vi "Amplitude Spectrum (sim).vi"() -> ()   [LabVIEW 2020]
doc: "Uses the FFT Spectrum (Mag-Phase) VI to window the signal and display the Amplitude and Phase spectrum. The example also uses the different averaging modes. A subVI simulates a sampled signal."
uses:
  <vilib>/measure/maspectr.llb/FFT Spectrum (Mag-Phase).vi
  <vilib>/measure/NI_MAPro.lvlib
panel:
  in  "sampling info":cluster{"Fs":dbl, "#s":dbl}={"Fs"=51200.0, "#s"=1024.0} {"#s" format="%#.6g"; "Fs" format="%#.6g"}
  in  "signal generator":T1={"type"=enum."Sine Wave", "frequency"=1000.0, "amplitude"=1.0}
  out "averages completed":dbl
  out "Linear averaging done":bool
  in  "Restart averaging":bool
  out "Phase spectrum":cluster{"f0":dbl, "df":dbl, "phase":dbl[]}(graph)
  in  "averaging parameters":T2={"averaging mode"=enum."RMS averaging", "weighting mode"=enum."Exponential", "number of averages"=10} {"number of averages" min=1}
  in  "window":T3(ring)=enum."Hanning"
  out "Amplitude spectrum":cluster{"f0":dbl, "df":dbl, "magnitude":dbl[]}(graph)
  in  "Stop":bool
  # "Overview: Demonstrates using the FFT Spectrum (Mag-Phase) VI to window the signal and display the Amplitude and Phase spectrum.\nRequirements: LabVIEW Full Development System\nInstructions: \n1. Run the VI.\n2. Change the signal generator type, frequency, and amplitude.\n3. Change the averaging parameters to explore various FFT averaging and weighting modes.\n4. Click Stop to stop the VI."
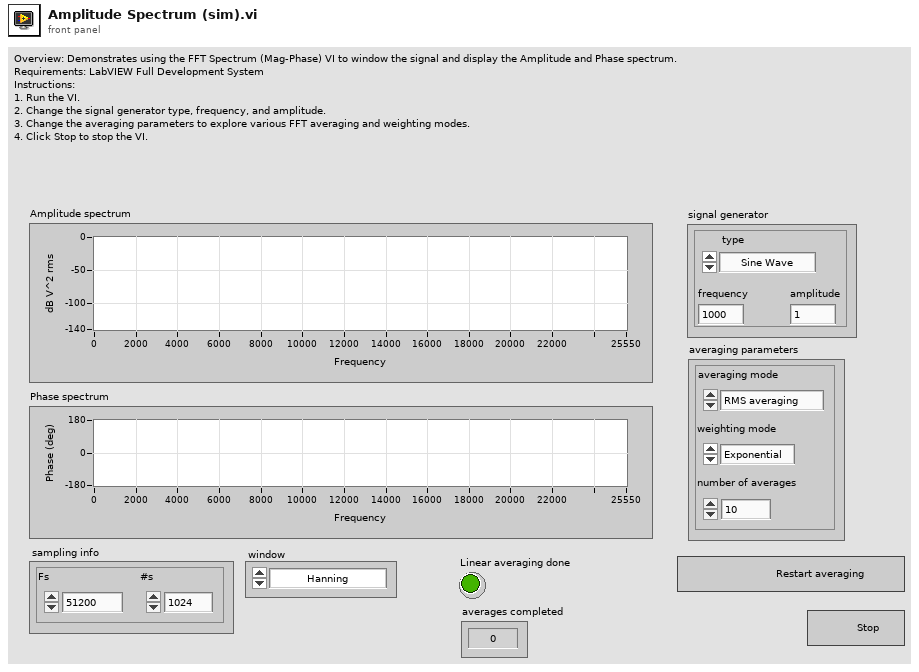
[diagram p1: front panel]
types:
  T1 = cluster{"type":enum16{"Sine Wave", "Triangle Wave", "Square Wave", "Sawtooth Wave"}, "frequency":dbl, "amplitude":dbl}
  T2 = cluster{"averaging mode":enum16{"No averaging", "Vector averaging", "RMS averaging", "Peak hold"}, "weighting mode":enum16{"Linear", "Exponential"}, "number of averages":u32}
  T3 = enum16{"None ", "Hanning", "Hamming", "Blackman-Harris", "Exact Blackman", "Blackman", "Flat Top", "4 Term B-Harris ", "7 Term B-Harris", "Low Sidelobe"}
  T4 = cluster{"dB On (F)":bool, "unwrap phase (F)":bool, "convert to degree (F)":bool}
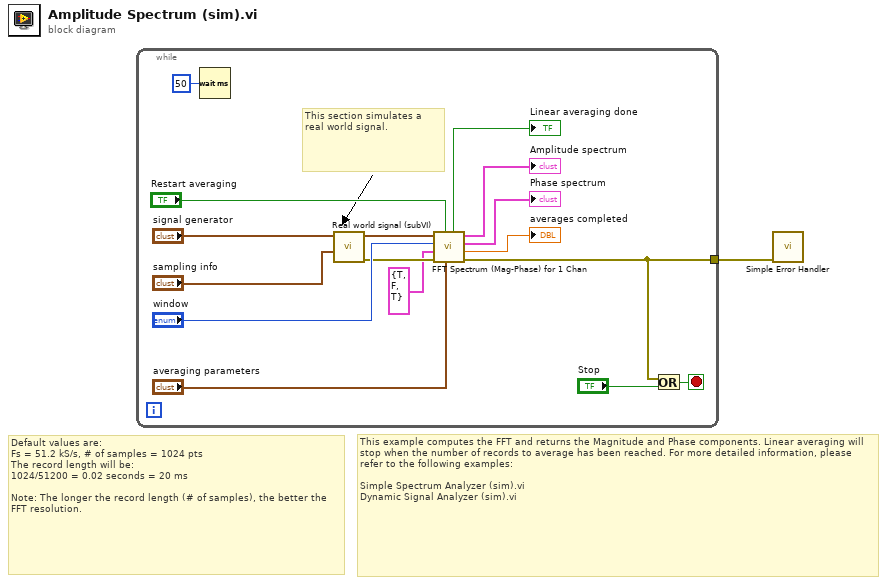
[diagram p0: block diagram]
diagram:
  # "This example computes the FFT and returns the Magnitude and Phase components. Linear averaging will stop when the number of records to average has been reached. For more detailed information, please refer to the following examples:\n\nSimple Spectrum Analyzer (sim).vi\nDynamic Signal Analyzer (sim).vi"
  # "Default values are:\nFs = 51.2 kS/s, # of samples = 1024 pts\nThe record length will be:\n1024/51200 = 0.02 seconds = 20 ms\n\nNote: The longer the record length (# of samples), the better the FFT resolution."
  n1 = while {
    tunnel: [w6] -> w1
    stop <- w7 stop-if-true
    # "This section simulates a real world signal."
    n2 = Wait (ms)(milliseconds to wait=u32 50 ("millisecond multiple")) -> ()  [unwired: 1 out]
    n3 = call "Real world signal (subVI).vi"("sampling info"="sampling info", "signal generator"="signal generator") -> ("error out"=w10:errorcluster, "time signal"=w5:waveform(dbl))  [unwired: 8 in]
    n4 = call-poly <vilib>:"FFT Spectrum (Mag-Phase) for 1 Chan.vi"("averaging parameters"="averaging parameters", "restart averaging (F)"="Restart averaging", "error in (no error)"=w10, "view"=T4 {"dB On (F)"=TRUE, "unwrap phase (F)"=FALSE, "convert to degree (F)"=TRUE}, "window"="window", "time signal"=w5) -> ("error out"=w6:errorcluster, "averages completed"=→"averages completed":dbl, "phase"=→"Phase spectrum":cluster{"f0":dbl, "df":dbl, "phase":dbl[]}, "magnitude"=→"Amplitude spectrum":cluster{"f0":dbl, "df":dbl, "magnitude":dbl[]}, "averaging done"=→"Linear averaging done":bool)  [unwired: 1 in]
    n5 = Or(x=w6, y="Stop") -> (x .or. y?=w7:bool)
  }
  n6 = call <vilib>:"Simple Error Handler.vi"("error in (no error)"=w1) -> ()  [unwired: 4 in, 5 out]
